vi "AtoDSigConvert.vi"(0 "Samples":dbl, 1 "Array Input":dbl[](array[numeric])) -> (2 "sCnSu32":u32[](array[numeric]), 3 "sCnSu16":u16[](array[numeric]), 4 "sCnSu8":u8[](array[numeric]))   [LabVIEW 2010]
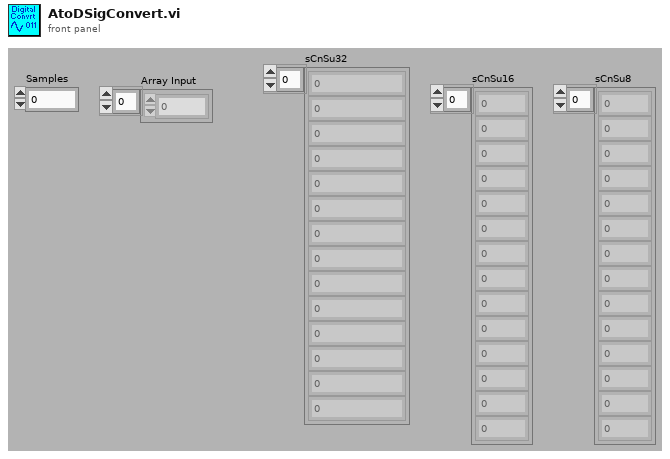
[diagram p1: front panel]
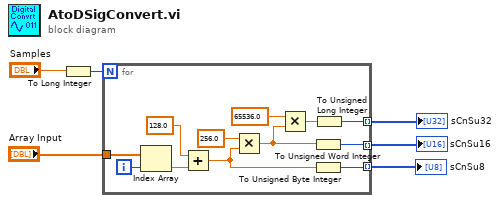
[diagram p0: block diagram]
diagram:
  n1 = To Long Integer(number="Samples") -> (32bit integer=w3:i32)
  n2 = for {
    N: w3 -> [_]
    tunnel: "Array Input" -> [w17]
    tunnel: [w14] -> w6 mode=indexing
    tunnel: [w16] -> w5 mode=indexing
    tunnel: [w10] -> w4 mode=indexing
    i -> [w18]
    n3 = Index Array(array=w17, index=w18) -> (element=w9:dbl)
    n4 = Add(x=128.0, y=w9) -> (x+y=w8:dbl)
    n5 = Multiply(x=256.0, y=w8) -> (x*y=w12:dbl)
    n6 = Multiply(x=65536.0, y=w12) -> (x*y=w13:dbl)
    n7 = To Unsigned Word Integer(number=w12) -> (unsigned 16bit integer=w16:u16)
    n8 = To Unsigned Byte Integer(number=w8) -> (unsigned 8bit integer=w14:u8)
    n9 = To Unsigned Long Integer(number=w13) -> (unsigned 32bit integer=w10:u32)
  }
  "sCnSu16" <- w5
  "sCnSu8" <- w6
  "sCnSu32" <- w4
